vi "GotoTables(aligned).vi"(0 "VRN IN":refnum<visa-resource-name>, 5 "Pulse Y":i32 min=-1000000 max=1000000, 7 "Pulse X":i32 min=-1000000 max=1000000, 9 "Pulse Z":i32 min=-1000000 max=1000000, 11 "Pulse P":i32 min=-1000000 max=1000000, 12 "Low Speed":u32=200 min=1 max=500000, 13 "High Speed":u32=30000 min=1 max=500000, 14 "Acceleration Time":u32=200 max=1000) -> (4 "VRN OUT":refnum<visa-resource-name>, 8 "OK Done":bool, 15 "error OUT":errorcluster)   [LabVIEW 2011]
uses:
  Globals.vi
panel:
  # "Sample program to show how to control Mark202/Mark204 Stage controller."
  # "1er caractère: X -> Erreur de commande\n                        K -> Commande bien reçue\n2e caractère:  L,M,W,# -> Erreur à l'arrêt\n                        K -> Arrêt normal\n3e caractère: R -> Prêt\n                       B -> Occupé"
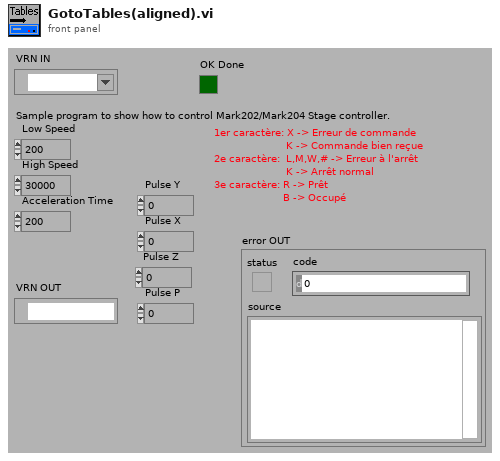
[diagram p1: front panel]
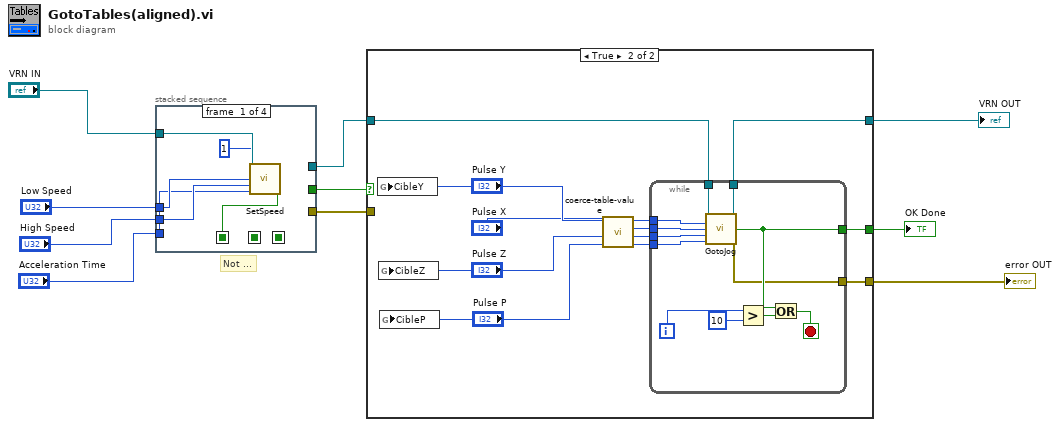
[diagram p0: block diagram]
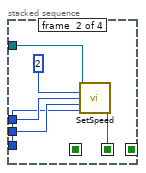
[diagram p2: hidden frame]
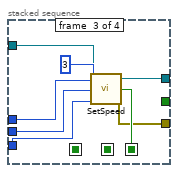
[diagram p3: hidden frame]
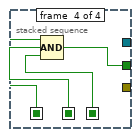
[diagram p4: hidden frame]
diagram:
  # "Not ..."
  n1 = stacked-sequence {
    seq-local: [w11 _ _ _] -> [_ _ _ w33]
    seq-local: [_ w17 _ _] -> [_ _ _ w32]
    seq-local: [_ _ w25 _] -> [_ _ _ w31]
    tunnel: "VRN IN" -> [w16 w22 w24 _]
    tunnel: [_ _ _ w30] -> w10
    tunnel: "Low Speed" -> [w15 w21 w29 _]
    tunnel: "High Speed" -> [w14 w20 w28 _]
    tunnel: "Acceleration Time" -> [w13 w19 w27 _]
    tunnel: [_ _ w24 _] -> w4
    tunnel: [_ _ w23 _] -> w1
    frame #0 {
      n2 = call "SetSpeed.vi"("VRN IN"=w16, "Axis Number"=u8 1, "Low Speed"=w15, "High Speed"=w14, "Acceleration Time"=w13) -> ("OK Done"=w11:bool)  [unwired: 8 in, 2 out]
    }
    frame #1 {
      n3 = call "SetSpeed.vi"("VRN IN"=w22, "Axis Number"=u8 2, "Low Speed"=w21, "High Speed"=w20, "Acceleration Time"=w19) -> ("OK Done"=w17:bool)  [unwired: 8 in, 2 out]
    }
    frame #2 {
      n4 = call "SetSpeed.vi"("VRN IN"=w24, "Axis Number"=u8 3, "Low Speed"=w29, "High Speed"=w28, "Acceleration Time"=w27) -> ("OK Done"=w25:bool, "error out"=w23:errorcluster)  [unwired: 8 in, 1 out]
    }
    frame #3 {
      n5 = Compound Arithmetic op=AND(w33, w32, w31) -> (w30:bool)
    }
  }
  n6 = case shown="True" w10 {
    selector: w10 -> [w36 _]
    tunnel: [w36 w48] -> w6
    tunnel: w4 -> [w35 w39]
    tunnel: [w35 w38] -> w3
    tunnel: [w34 w37] -> w2
    tunnel: w1 -> [w34 _]
    frame False {
    }
    frame True {
      n7 = global write "Globals.vi" "CibleY"("Pulse Y") -> ()
      n8 = global write "Globals.vi" "CibleZ"("Pulse Z") -> ()
      n9 = global write "Globals.vi" "CibleP"("Pulse P") -> ()
      n10 = call "coerce-table-value.vi"("Y"="Pulse Y", "X"="Pulse X", "Z"="Pulse Z", "P"="Pulse P") -> ("coerced Y"=w47:i32, "coerced X"=w46:i32, "coerced Z"=w45:i32, "coerced P"=w44:i32)  [unwired: 1 out]
      n11 = while {
        tunnel: w39 -> [w60]
        tunnel: [w51] -> w48
        tunnel: w47 -> [w59]
        tunnel: w46 -> [w58]
        tunnel: w45 -> [w57]
        tunnel: w44 -> [w56]
        tunnel: [w50] -> w38
        tunnel: [w49] -> w37
        i -> [w53]
        stop <- w55 stop-if-true
        n12 = call "GotoJog.vi"("reference"=w60, "Position Y"=w59, "Position X"=w58, "Position Z"=w57, "Position F"=w56) -> ("reference dup"=w50:refnum<visa-resource-name>, "OK Done"=w51:bool, "error OUT"=w49:errorcluster)  [unwired: 8 in]
        n13 = Greater?(x=w53, y=10) -> (0:w54:bool)
        n14 = Or(x=w51, y=w54) -> (x .or. y?=w55:bool)
      }
    }
  }
  "OK Done" <- w6
  "VRN OUT" <- w3
  "error OUT" <- w2
